vi "Event Driven Data Transfer.vi"() -> ()   [LabVIEW 2013]
uses:
  lightfield-automation-labview/LightField Automation.lvclass
panel:
  in  "ExperimentName":string
  out "Intensity Graph":dbl[][](graph)
  out "Time Per Loop":dbl
  out "Waveform Graph":dbl[](graph)
  out "# elements in queue":i32
  in  "stop":bool
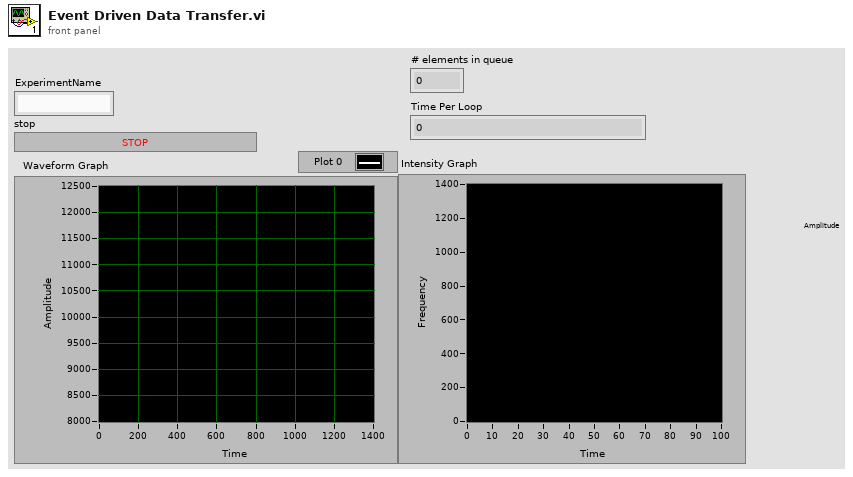
[diagram p1: front panel]
types:
  T1 = cluster{"Image":dbl[][][], "Frame Size":cluster{"F":i32, "Y":i32, "X":i32}}[]
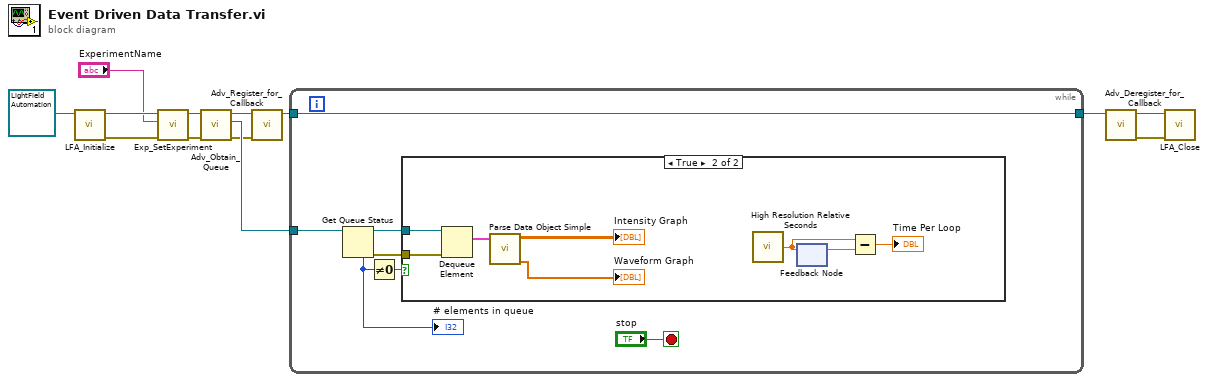
[diagram p0: block diagram]
diagram:
  n1 = call "LFA_Initialize.vi"("LightField Automation in"=refnum<class "LightField Automation.lvclass"> refnum ("LightField Automation.lvclass")) -> ("error out"=w5:errorcluster, "LightField Automation out"=w7:refnum<class "LightField Automation.lvclass">)  [unwired: 9 in]
  n2 = call "Exp_SetExperiment.vi"("error in (no error)"=w5, "ExperimentName"="ExperimentName", "LightField Automation in"=w7) -> ("error out"=w4:errorcluster, "LightField Automation out"=w6:refnum<class "LightField Automation.lvclass">)  [unwired: 7 in]
  n3 = call "Adv_Obtain_Queue.vi"("error in (no error)"=w4, "LightField Automation in"=w6) -> ("error out"=w11:errorcluster, "Queue Reference"=w12:refnum<queue>, "LightField Automation out"=w13:refnum<class "LightField Automation.lvclass">)  [unwired: 7 in]
  n4 = call "Adv_Register_for_Callback.vi"("error in (no error)"=w11, "LightField Automation in"=w13) -> ("LightField Automation out"=w10:refnum<class "LightField Automation.lvclass">)  [unwired: 8 in, 1 out]
  n5 = while {
    tunnel: w12 -> [w19]
    tunnel: w10 -> [w14]
    tunnel: [w14] -> w9
    stop <- "stop" stop-if-true
    n6 = Get Queue Status(queue=w19) -> (queue out=w18:refnum<queue>, error out=w17:errorcluster, # elements in queue=w15:i32)  [unwired: 2 in, 5 out]
    "# elements in queue" <- w15
    n7 = Not Equal To 0?(x=w15) -> (x != 0?=w16:bool)
    n8 = case shown="True" w16 {
      tunnel: w18 -> [_ w28]
      tunnel: w17 -> [_ w27]
      frame False {
      }
      frame True {
        n9 = Dequeue Element(queue=w28, error in (no error)=w27) -> (element=w23:T1)  [unwired: 1 in, 3 out]
        n10 = call "Parse Data Object Simple.vi"("Data"=w23) -> ("ROI 1, Frame 1, Row 1"=→"Waveform Graph":dbl[], "ROI 1, Frame 1"=→"Intensity Graph":dbl[][])  [unwired: 9 in]
        n11 = call <vilib>:"High Resolution Relative Seconds.vi"() -> ("relative seconds"=w25:dbl)
        n12 = feedback-in #1(w25) -> ()
        n13 = feedback #1() -> (w26:dbl)  [unwired: 1 in]
        n14 = Subtract(x=w25, y=w26) -> (x-y=→"Time Per Loop":dbl)
      }
    }
  }
  n15 = call "Adv_Deregister_for_Callback.vi"("LightField Automation in"=w9) -> ("error out"=w2:errorcluster, "LightField Automation out"=w1:refnum<class "LightField Automation.lvclass">)  [unwired: 9 in]
  n16 = call "LFA_Close.vi"("error in (no error)"=w2, "LightField Automation in"=w1) -> ()  [unwired: 8 in, 2 out]
